vi "Position Conversion.vi"(0 "Child Hwnd":u32, 5 "Parent Position":T2, 11 "error in (no error)":errorcluster) -> (6 "Child Position":T1, 15 "error out":errorcluster)   [LabVIEW 2016, in "LV MDI.lvclass"]
uses:
  LV MDI.lvclass
  protected/Offset.ctl
  protected/Postion.ctl
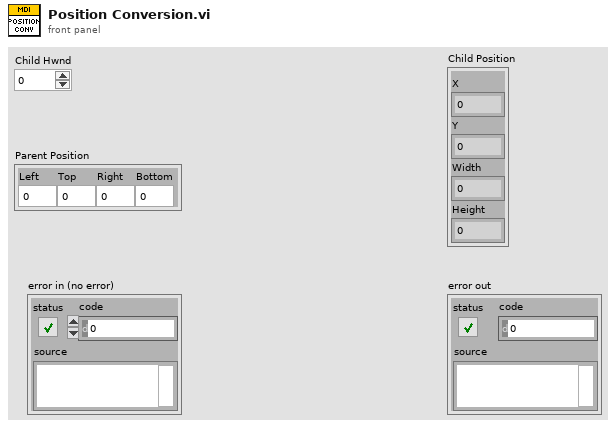
[diagram p1: front panel]
types:
  T1 = typedef "LV MDI.lvclass/Postion.ctl" = cluster{"X":i32, "Y":i32, "Width":i32, "Height":i32}
  T2 = typedef "LV MDI.lvclass/Offset.ctl" = cluster{"Left":i32, "Top":i32, "Right":i32, "Bottom":i32}
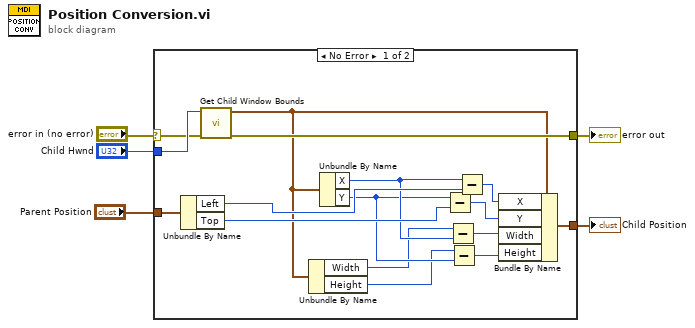
[diagram p0: block diagram]
diagram:
  n1 = case shown="No Error" "error in (no error)" {
    selector: "error in (no error)" -> [w15 w22]
    tunnel: "Parent Position" -> [w19 _]
    tunnel: [w18 _] -> w4
    tunnel: "Child Hwnd" -> [w17 _]
    tunnel: [w16 w22] -> w2
    frame No Error {
      n2 = Unbundle By Name(w19) -> ("Left"=w20:i32, "Top"=w21:i32)
      n3 = call "Get Child Window Bounds.vi"("error in (no error)"=w15, "Child Hwnd"=w17) -> ("error out"=w16:errorcluster, "lpRect"=w8:T1)  [unwired: 8 in]
      n4 = Unbundle By Name(w8) -> ("Width"=w7:i32, "Height"=w6:i32)
      n5 = Unbundle By Name(w8) -> ("X"=w12:i32, "Y"=w9:i32)
      n6 = Subtract(x=w9, y=w21) -> (x-y=w11:i32)
      n7 = Subtract(x=w7, y=w12) -> (x-y=w13:i32)
      n8 = Subtract(x=w6, y=w9) -> (x-y=w10:i32)
      n9 = Subtract(x=w12, y=w20) -> (x-y=w14:i32)
      n10 = Bundle By Name(cluster=w8, "X"=w14, "Y"=w11, "Width"=w13, "Height"=w10) -> (w18:T1)
    }
    frame Error {
    }
  }
  "Child Position" <- w4
  "error out" <- w2
